vi "UE9 eAIN Example.vi"() -> (0 "error out":errorcluster)   [LabVIEW 2021]
panel:
  in  "AIN Range":u16(ring) items=["LJ_rgBIP5V", "LJ_rgUNI5V", "LJ_rgUNI2P5V", "LJ_rgUNI1P25V", "LJ_rgUNIP625V"]
  in  "Resolution":i32=12
  in  "FirstFound":bool=TRUE
  in  "ConnectionType":u16(ring) items=["LJ_ctUSB", "LJ_ctETHERNET"]
  in  "Address":string="192.168.1.209"
  in  "Channel":i32
  out "Error Message":string
  out "Value Read":dbl format="%.9f"
  # "Reads 1 analog input using the UD easy function eAIN."
  # "Specify an IP address for Ethernet, or Local ID\nfor USB.  If FirstFound is selected, Local ID is\nignored for USB."
  # "14 = Vref\n15 = GND\n132 = Vsupply\n133 = Temp K"
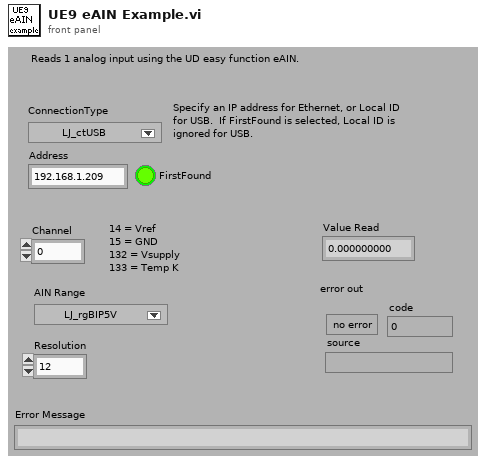
[diagram p1: front panel]
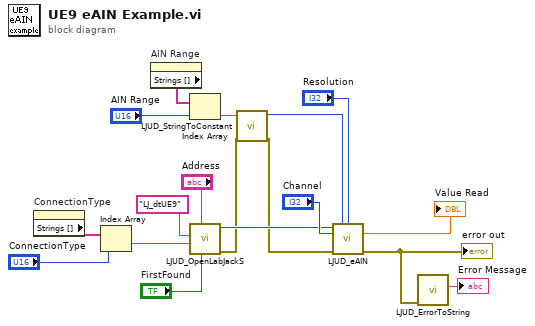
[diagram p0: block diagram]
diagram:
  n1 = property on="ConnectionType" class="Ring (strict)"() -> ("Strings []"=w8:string[])  [unwired: 2 in, 2 out]
  n2 = Index Array(array=w8, index="ConnectionType") -> (element=w13:string)
  n3 = property on="AIN Range" class="Ring (strict)"() -> ("Strings []"=w3:string[])  [unwired: 2 in, 2 out]
  n4 = Index Array(array=w3, index="AIN Range") -> (element=w1:string)
  n5 = call "LJUD_OpenLabJackS.vi"("FirstFound"="FirstFound", "Address"="Address", "ConnectionType"=w13, "DeviceType"="LJ_dtUE9") -> ("error out"=w5:errorcluster, "Handle"=w11:i32)  [unwired: 5 in, 1 out]
  n6 = call "LJUD_StringToConstant.vi"("error in"=w5, "String"=w1) -> ("error out"=w4:errorcluster, "Constant Number"=w7:i32)  [unwired: 8 in]
  n7 = call "LJUD_eAIN.vi"("Handle In"=w11, "Range"=w7, "Resolution"="Resolution", "ChannelP"="Channel", "error in"=w4) -> ("Voltage"=→"Value Read":dbl, "error out"=w17:errorcluster)  [unwired: 8 in, 1 out]
  "error out" <- w17
  n8 = call "LJUD_ErrorToString.vi"("error in"=w17) -> ("String"=→"Error Message":string)  [unwired: 10 in]
